vi "Serialization.vi"() -> ()   [LabVIEW 2012]
panel:
  in  "conversion type":bool
  out "data out":T1
  in  "text":string
  in  "data in":T1={"number"=123.456, "string"="quick brown fox", "path"=path "foo/bar/baz.vi", "array"=[enum."baz", enum."foo", enum."bar"], "sub cluster"={"Boolean"=TRUE, "int"=42}}
  # "Converting LabVIEW data to/from text can be used for exporting/importing readable/editable configuration files\nor for easy text formatting of compound data (e.g. when throwing an error or writing to a log file)."
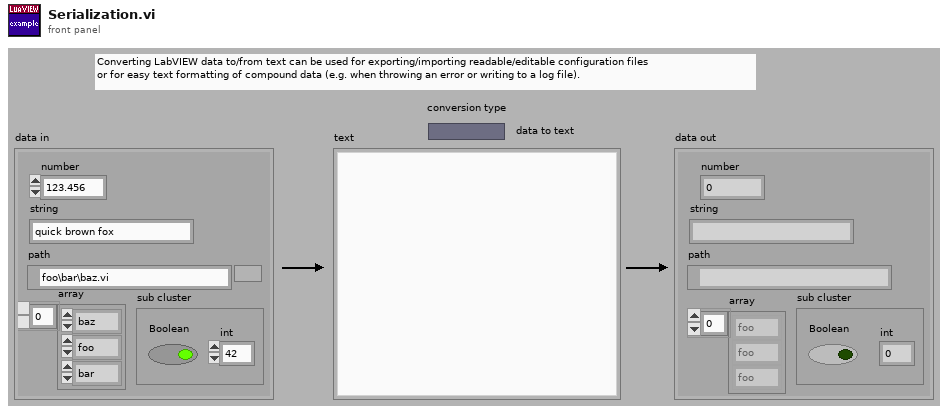
[diagram p1: front panel]
types:
  T1 = cluster{"number":dbl, "string":string, "path":path, "array":enum16{"foo", "bar", "baz"}[], "sub cluster":cluster{"Boolean":bool, "int":u32}}
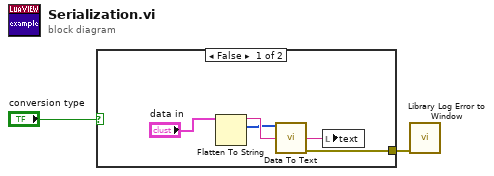
[diagram p0: block diagram]
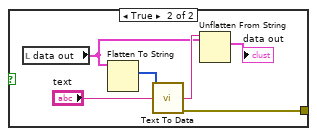
[diagram p2: hidden frame]
diagram:
  n1 = case shown="False" "conversion type" {
    tunnel: [w4 w8] -> w2
    frame False {
      n2 = Flatten To String(anything="data in") -> (data string=w5:string, type string=w3:i16[])  [unwired: 3 in, 1 out]
      n3 = call "Data To Text.vi"("type descriptor"=w3, "flat data"=w5) -> ("text"=w7:string, "error out"=w4:errorcluster)  [unwired: 12 in]
      n4 = local write "text"(w7) -> ()
    }
    frame True {
      n5 = local read "data out"() -> (w11:T1)
      n6 = Flatten To String(anything=w11) -> (type string=w10:i16[])  [unwired: 3 in, 2 out]
      n7 = call "Text To Data.vi"("type descriptor"=w10, "text"="text") -> ("flat data"=w13:string, "error out"=w8:errorcluster)  [unwired: 12 in]
      n8 = Unflatten From String(type=w11, binary string=w13) -> (value=→"data out":T1)  [unwired: 3 in, 2 out]
    }
  }
  n9 = call "Library Log Error to Window.vi"("error in (no error)"=w2) -> ()  [unwired: 13 in, 2 out]
